vi "NoiseFloor_LowPass.vi"(9 "s_axis_data_tdata":fxp<+/-,16,1>, 10 "s_axis_data_tvalid":bool) -> (1 "m_axis_data_tdata":fxp<+/-,24,5>, 2 "m_axis_data_tvalid":bool, 3 "s_axis_data_tready":bool)   [LabVIEW 2018]
uses:
  <vilib>/rvi/IPIntegrationNode/IPINode_Typedef/niFpgaIPINodeSupportedFamilies.ctl
  <vilib>/rvi/IPIntegrationNode/IPINode_Utilities/niFpgaIPINodeSimCore.vi
  <vilib>/rvi/XilinxIP/XIPIN_XNode/niFpgaXIPIN.xnode
  DigitalFilterDesign/FIR_Filter_Configuration/FIR Compiler/xsim.dir/FIR_Compiler_3CE652926F5B43F18022D1349C670FA0/xsimk_3CE652926F5B43F18022D1349C670FA0.dll
  <vilib>/rvi/IPIntegrationNode/IPINode_Xnode/niFpgaIPINode.xnode
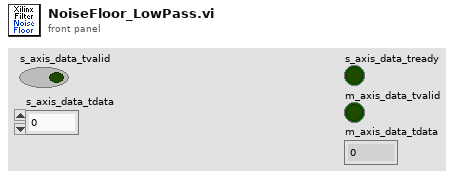
[diagram p1: front panel]
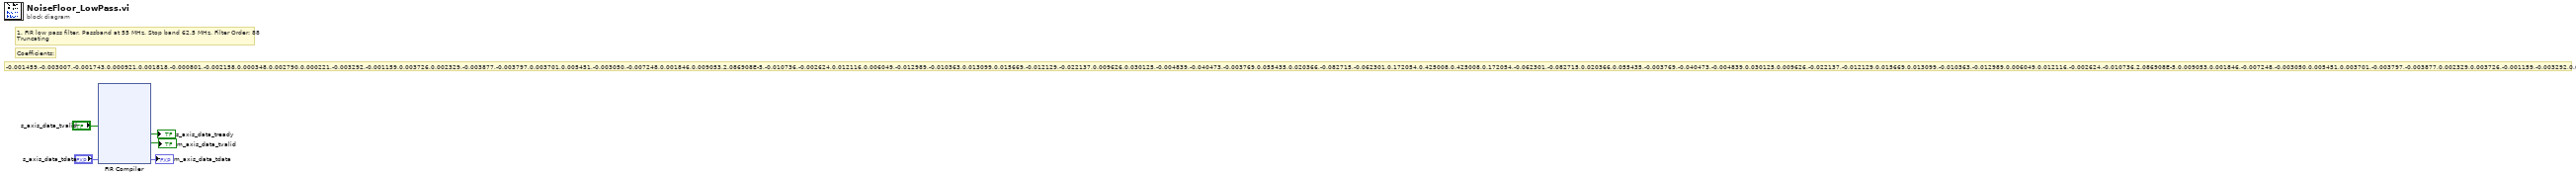
[diagram p0: block diagram]
diagram:
  # "-0.001459,-0.003007,-0.001743,0.000921,0.001818,-0.000801,-0.002158,0.000348,0.002790,0.000221,-0.003292,-0.001159,0.003726,0.002329,-0.003877,-0.003797,0.003701,0.005451,-0.003050,-0.007248,0.001846,0.009053,2.086908E-5,-0.010736,-0.002624,0.012116,0.006049,-0.012989,-0.010363,0.013099,0.015669,-0.012129,-0.022137,0.009626,0.030125,-0.004839,-0.040473,-0.003769,0.055435,0.020366,-0.082715,-0.062301,0.172054,0.425008,0.425008,0.172054,-0.062301,-0.082715,0.020366,0.055435,-0.003769,-0.040473,-0.004839,0.030125,0.009626,-0.022137,-0.012129,0.015669,0.013099,-0.010363,-0.012989,0.006049,0.012116,-0.002624,-0.010736,2.086908E-5,0.009053,0.001846,-0.007248,-0.003050,0.005451,0.003701,-0.003797,-0.003877,0.002329,0.003726,-0.001159,-0.003292,0.000221,0.002790,0.000348,-0.002158,-0.000801,0.001818,0.000921,-0.001743,-0.003007,-0.001459"
  # "Coefficients:"
  # "1.\tFIR low pass filter. Passband at 55 MHz. Stop band 62.5 MHz. Filter Order: 88 \nTruncating"
  n1 = xnode ("FIR Compiler")("s_axis_data_tvalid"="s_axis_data_tvalid", "s_axis_data_tdata"="s_axis_data_tdata") -> ("s_axis_data_tready"=→"s_axis_data_tready":bool, "m_axis_data_tvalid"=→"m_axis_data_tvalid":bool, "m_axis_data_tdata"=→"m_axis_data_tdata":fxp<+/-,24,5>)
